vi "Func-엑셀 데이터를 그래프로 출력.vi"() -> ()   [LabVIEW 2015] (continued)
45\t45\t48.154\n45\t45\t48.16\n45\t45\t48.165\n45\t45\t48.164\n45\t45\t48.166\n45\t45\t48.17\n45\t45\t48.174\n45\t45\t48.179\n45\t45\t48.186\n45\t45\t48.187\n45\t45\t48.193\n45\t45\t48.198\n45\t45\t48.202\n45\t45\t48.205\n45\t45\t48.21\n45\t45\t48.216\n45\t45\t48.22\n45\t45\t48.222\n45\t45\t48.229\n45\t45\t48.232\n45\t45\t48.238\n45\t45\t48.24\n45\t45\t48.243\n45\t45\t48.246\n45\t45\t48.248\n45\t45\t48.252\n45\t45\t48.255\n45\t45\t48.258\n45\t45\t48.265\n45\t45\t48.273\n45\t45\t48.283\n45\t45\t48.288\n45\t45\t48.292\n45\t45\t48.296\n45\t45\t48.298\n45\t45\t48.302\n45\t45\t48.299\n45\t45\t48.305\n45\t45\t48.31\n45\t45\t48.314\n45\t45\t48.322\n45\t45\t48.323\n45\t45\t48.325\n45\t45\t48.329\n45\t45\t48.329\n45\t45\t48.334\n45\t45\t48.339\n45\t45\t48.344\n45\t45\t48.352\n45\t45\t48.359\n45\t45\t48.364\n45\t45\t48.366\n45\t45\t48.369\n45\t45\t48.374\n45\t45\t48.375\n45\t45\t48.382\n45\t45\t48.384\n45\t45\t48.39\n45\t45\t48.395\n45\t45\t48.393\n45\t45\t48.397\n45\t45\t48.402\n45\t45\t48.409\n45\t45\t48.417\n45\t45\t48.421\n45\t45\t48.427\n45\t45\t48.431\n45\t45\t48.434\n45\t45\t48.439\n45\t45\t48.441\n45\t45\t48.444\n45\t45\t48.446\n45\t45\t48.449\n45\t45\t48.454\n45\t45\t48.454\n45\t45\t48.46\n45\t45\t48.462\n45\t45\t48.47\n45\t45\t48.479\n45\t45\t48.481\n45\t45\t48.488\n45\t45\t48.491\n45\t45\t48.495\n45\t45\t48.494\n45\t45\t48.495\n45\t45\t48.497\n45\t45\t48.496\n45\t45\t48.503\n45\t45\t48.509\n45\t45\t48.513\n45\t45\t48.518\n45\t45\t48.521\n45\t45\t48.53\n45\t45\t48.531\n45\t45\t48.533\n45\t45\t48.539\n45\t45\t48.543\n45\t45\t48.546\n45\t45\t48.55\n45\t45\t48.552\n45\t45\t48.554\n45\t45\t48.557\n45\t45\t48.562\n45\t45\t48.567\n45\t45\t48.571\n45\t45\t48.577\n45\t45\t48.58\n45\t45\t48.582\n45\t45\t48.59\n45\t45\t48.592\n45\t45\t48.597\n45\t45\t48.596\n45\t45\t48.598\n45\t45\t48.605\n45\t45\t48.605\n45\t45\t48.606\n45\t45\t48.607\n45\t45\t48.617\n45\t45\t48.624\n45\t45\t48.627\n45\t45\t48.631\n45\t45\t48.638\n45\t45\t48.646\n45\t45\t48.646\n45\t45\t48.649\n45\t45\t48.656\n45\t45\t48.66\n45\t45\t48.663\n45\t45\t48.667\n45\t45\t48.673\n45\t45\t48.677\n45\t45\t48.678\n45\t45\t48.68\n45\t45\t48.679\n45\t45\t48.682\n45\t45\t48.683\n45\t45\t48.689\n45\t45\t48.691\n45\t45\t48.694\n45\t45\t48.7\n45\t45\t48.7\n45\t45\t48.703\n45\t45\t48.709\n45\t45\t48.713\n45\t45\t48.716\n45\t45\t48.725\n45\t45\t48.729\n45\t45\t48.732\n45\t45\t48.734\n45\t45\t48.739\n45\t45\t48.743\n45\t45\t48.746\n45\t45\t48.747\n45\t45\t48.753\n45\t45\t48.761\n45\t45\t48.762\n45\t45\t48.767\n45\t45\t48.767\n45\t45\t48.774\n45\t45\t48.779\n45\t45\t48.778\n45\t45\t48.782\n45\t45\t48.789\n45\t45\t48.789\n45\t45\t48.79\n45\t45\t48.793\n45\t45\t48.801\n45\t45\t48.802\n45\t45\t48.808\n45\t45\t48.812\n45\t45\t48.816\n45\t45\t48.82\n45\t45\t48.821\n45\t45\t48.826\n45\t45\t48.825\n45\t45\t48.83\n45\t45\t48.829\n45\t45\t48.829\n45\t45\t48.83\n45\t45\t48.834\n45\t45\t48.837\n45\t45\t48.839\n45\t45\t48.846\n45\t45\t48.853\n45\t45\t48.859\n45\t45\t48.862\n45\t45\t48.869\n45\t45\t48.875\n45\t45\t48.881\n45\t45\t48.882\n45\t45\t48.884\n45\t45\t48.891\n45\t45\t48.89\n45\t45\t48.891\n45\t45\t48.892\n45\t45\t48.895\n45\t45\t48.896\n45\t45\t48.903\n45\t45\t48.905\n45\t45\t48.909\n45\t45\t48.913\n45\t45\t48.92\n45\t45\t48.926\n45\t45\t48.927\n45\t45\t48.931\n45\t45\t48.932\n45\t45\t48.939\n45\t45\t48.939\n45\t45\t48.941\n45\t45\t48.942\n45\t45\t48.949\n45\t45\t48.955\n45\t45\t48.957\n45\t45\t48.963\n45\t45\t48.965\n45\t45\t48.975\n45\t45\t48.979\n45\t45\t48.982\n45\t45\t48.987\n45\t45\t48.988\n45\t45\t48.994\n45\t45\t48.995\n45\t45\t48.991\n45\t45\t48.992\n45\t45\t48.993\n45\t45\t48.996\n45\t45\t48.999\n45\t45\t49.003\n45\t45\t49.007\n45\t45\t49.015\n45\t45\t49.02\n45\t45\t49.025\n45\t45\t49.028\n45\t45\t49.033\n45\t45\t49.036\n45\t45\t49.037\n45\t45\t49.042\n45\t45\t49.045\n45\t45\t49.05\n45\t45\t49.051\n45\t45\t49.055\n45\t45\t49.059\n45\t45\t49.059\n45\t45\t49.057\n45\t45\t49.058\n45\t45\t49.058\n45\t45\t49.061\n45\t45\t49.064\n45\t45\t49.069\n45\t45\t49.073\n45\t45\t49.077\n45\t45\t49.084\n45\t45\t49.086\n45\t45\t49.093\n45\t45\t49.095\n45\t45\t49.101\n45\t45\t49.105\n45\t45\t49.109\n45\t45\t49.111\n45\t45\t49.115\n45\t45\t49.12\n45\t45\t49.12\n45\t45\t49.123\n45\t45\t49.125\n45\t45\t49.131\n45\t45\t49.132\n45\t45\t49.134\n45\t45\t49.139\n45\t45\t49.142\n45\t45\t49.146\n45\t45\t49.148\n45\t45\t49.151\n45\t45\t49.154\n45\t45\t49.159\n45\t45\t49.161\n45\t45\t49.162\n45\t45\t49.165\n45\t45\t49.166\n45\t45\t49.171\n45\t45\t49.173\n45\t45\t49.177\n45\t45\t49.179\n45\t45\t49.184\n45\t45\t49.189\n45\t45\t49.189\n45\t45\t49.195\n45\t45\t49.194\n45\t45\t49.196\n45\t45\t49.199\n45\t45\t49.196\n45\t45\t49.201\n45\t45\t49.204\n45\t45\t49.209\n45\t45\t49.218\n45\t45\t49.221\n45\t45\t49.227\n45\t45\t49.23\n45\t45\t49.232\n45\t45\t49.233\n45\t45\t49.229\n45\t45\t49.232\n45\t45\t49.234\n45\t45\t49.239\n45\t45\t49.241\n45\t45\t49.246\n45\t45\t49.254\n45\t45\t49.256\n45\t45\t49.257\n45\t45\t49.255\n45\t45\t49.259\n45\t45\t49.259\n45\t45\t49.266\n45\t45\t49.27\n45\t45\t49.271\n45\t45\t49.28\n45\t45\t49.282\n45\t45\t49.284\n45\t45\t49.287\n45\t45\t49.29\n45\t45\t49.296\n45\t45\t49.299\n45\t45\t49.301\n45\t45\t49.302\n45\t45\t49.303\n45\t45\t49.305\n45\t45\t49.31\n45\t45\t49.309\n45\t45\t49.311\n45\t45\t49.314\n45\t45\t49.316\n45\t45\t49.316\n45\t45\t49.317\n45\t45\t49.323\n45\t45\t49.327\n45\t45\t49.332\n45\t45\t49.337\n45\t45\t49.34\n45\t45\t49.344\n45\t45\t49.341\n45\t45\t49.343\n45\t45\t49.349\n45\t45\t49.35\n45\t45\t49.352\n45\t45\t49.355\n45\t45\t49.363\n45\t45\t49.365\n45\t45\t49.368\n45\t45\t49.371\n45\t45\t49.375\n45\t45\t49.379\n45\t45\t49.379\n45\t45\t49.384\n45\t45\t49.389\n45\t45\t49.391\n45\t45\t49.393\n45\t45\t49.399\n45\t45\t49.401\n45\t45\t49.405\n45\t45\t49.41\n45\t45\t49.411\n45\t45\t49.413\n45\t45\t49.412\n45\t45\t49.412\n45\t45\t49.413\n45\t45\t49.413\n45\t45\t49.415\n45\t45\t49.419\n45\t45\t49.423\n45\t45\t49.428\n45\t45\t49.433\n45\t45\t49.434\n45\t45\t49.439\n45\t45\t49.44\n45\t45\t49.443\n45\t45\t49.446\n45\t45\t49.45\n45\t45\t49.452\n45\t45\t49.455\n45\t45\t49.463\n45\t45\t49.464\n45\t45\t49.467\n45\t45\t49.466\n45\t45\t49.466\n45\t45\t49.466\n45\t45\t49.471\n45\t45\t49.472\n45\t45\t49.476\n45\t45\t49.479\n45\t45\t49.484\n45\t45\t49.488\n45\t45\t49.489\n45\t45\t49.495\n45\t45\t49.502\n45\t45\t49.507\n45\t45\t49.513\n45\t45\t49.515\n45\t45\t49.517\n45\t45\t49.517\n45\t45\t49.516\n45\t45\t49.517\n45\t45\t49.516\n45\t45\t49.521\n45\t45\t49.524\n45\t45\t49.526\n45\t45\t49.53\n45\t45\t49.531\n45\t45\t49.533\n45\t45\t49.536\n45\t45\t49.541\n45\t45\t49.545\n45\t45\t49.546\n45\t45\t49.552\n45\t45\t49.556\n45\t45\t49.557\n45\t45\t49.554\n45\t45\t49.554\n45\t45\t49.554\n45\t45\t49.555\n45\t45\t49.557\n45\t45\t49.561\n45\t45\t49.564\n45\t45\t49.57\n45\t45\t49.579\n45\t45\t49.582\n45\t45\t49.589\n45\t45\t49.588\n45\t45\t49.593\n45\t45\t49.598\n45\t45\t49.596\n45\t45\t49.599\n45\t45\t49.599\n45\t45\t49.604\n45\t45\t49.6\n45\t45\t49.601\n45\t45\t49.605\n45\t45\t49.605\n45\t45\t49.606\n45\t45\t49.608\n45\t45\t49.614\n45\t45\t49.617\n45\t45\t49.619\n45\t45\t49.623\n45\t45\t49.627\n45\t45\t49.629\n45\t45\t49.629\n45\t45\t49.633\n45\t45\t49.637\n45\t45\t49.638\n45\t45\t49.643\n45\t45\t49.644\n45\t45\t49.647\n45\t45\t49.653\n45\t45\t49.65\n45\t45\t49.654\n45\t45\t49.654\n45\t45\t49.657\n45\t45\t49.662\n45\t45\t49.661\n45\t45\t49.666\n45\t45\t49.664\n45\t45\t49.67\n45\t45\t49.672\n45\t45\t49.677\n45\t45\t49.679\n45\t45\t49.683\n45\t45\t49.689\n45\t45\t49.691\n45\t45\t49.693\n45\t45\t49.699\n45\t45\t49.702\n45\t45\t49.703\n45\t45\t49.705\n45\t45\t49.707\n45\t45\t49.709\n45\t45\t49.711\n45\t45\t49.714\n45\t45\t49.714\n45\t45\t49.716\n45\t45\t49.716\n45\t45\t49.721\n45\t45\t49.72\n45\t45\t49.722\n45\t45\t49.722\n45\t45\t49.725\n45\t45\t49.732\n45\t45\t49.734\n45\t45\t49.737\n45\t45\t49.738\n45\t45\t49.748\n45\t45\t49.75\n45\t45\t49.75\n45\t45\t49.751\n45\t45\t49.753\n45\t45\t49.755\n45\t45\t49.754\n45\t45\t49.756\n45\t45\t49.753\n45\t45\t49.756\n45\t45\t49.759\n45\t45\t49.763\n45\t45\t49.764\n45\t45\t49.767\n45\t45\t49.772\n45\t45\t49.777\n45\t45\t49.779\n45\t45\t49.779\n45\t45\t49.785\n45\t45\t49.788\n45\t45\t49.79\n45\t45\t49.788\n45\t45\t49.792\n45\t45\t49.799\n45\t45\t49.797\n45\t45\t49.799\n45\t45\t49.807\n45\t45\t49.81\n45\t45\t49.809\n45\t45\t49.807\n45\t45\t49.809\n45\t45\t49.81\n45\t45\t49.809\n45\t45\t49.811\n45\t45\t49.816\n45\t45\t49.821\n45\t45\t49.825\n45\t45\t49.828\n45\t45\t49.83\n45\t45\t49.832\n45\t45\t49.833\n45\t45\t49.834\n45\t45\t49.839\n45\t45\t49.84\n45\t45\t49.842\n45\t45\t49.843\n45\t45\t49.847\n45\t45\t49.853\n45\t45\t49.851\n45\t45\t49.854\n45\t45\t49.857\n45\t45\t49.859\n45\t45\t49.857\n45\t45\t49.857\n45\t45\t49.861\n45\t45\t49.864\n45\t45\t49.866\n45\t45\t49.869\n45\t45\t49.871\n45\t45\t49.878\n45\t45\t49.875\n45\t45\t49.878\n45\t45\t49.879\n45\t45\t49.88\n45\t45\t49.885\n45\t45\t49.886\n45\t45\t49.891\n45\t45\t49.893\n45\t45\t49.898\n45\t45\t49.903\n45\t45\t49.909\n45\t45\t49.909\n45\t45\t49.911\n45\t45\t49.916\n45\t45\t49.918\n45\t45\t49.918\n45\t45\t49.92\n45\t45\t49.92\n45\t45\t49.921\n45\t45\t49.92\n45\t45\t49.925\n45\t45\t49.927\n45\t45\t49.928\n45\t45\t49.932\n45\t45\t49.939\n45\t45\t49.943\n45\t45\t49.941\n45\t45\t49.941\n45\t45\t49.943\n45\t45\t49.943\n45\t45\t49.944\n45\t45\t49.945\n45\t45\t49.95\n45\t45\t49.952\n45\t45\t49.954\n45\t45\t49.956\n45\t45\t49.959\n45\t45\t49.96\n45\t45\t49.96\n45\t45\t49.963\n45\t45\t49.963\n45\t45\t49.965\n45\t45\t49.968\n45\t45\t49.97\n45\t45\t49.969\n45\t45\t49.973\n45\t45\t49.979\n45\t45\t49.981\n45\t45\t49.976\n45\t45\t49.98\n45\t45\t49.984\n45\t45\t49.986\n45\t45\t49.986\n45\t45\t49.987\n45\t45\t49.995\n45\t45\t49.992\n45\t45\t49.996\n45\t45\t49.999\n45\t45\t50.003\n45\t45\t50.009\n45\t45\t50.009\n45\t45\t50.013\n45\t45\t50.016\n45\t45\t50.014\n45\t45\t50.015\n45\t45\t50.014\n45\t45\t50.014\n45\t45\t50.017\n45\t45\t50.018\n45\t45\t50.022\n45\t45\t50.021\n45\t45\t50.024\n45\t45\t50.028\n45\t45\t50.029\n45\t45\t50.031\n45\t45\t50.035\n45\t45\t50.04\n45\t45\t50.044\n45\t45\t50.045\n45\t45\t50.049\n45\t45\t50.055\n45\t45\t50.054\n45\t45\t50.058\n45\t45\t50.059\n45\t45\t50.063\n45\t45\t50.066\n45\t45\t50.063\n45\t45\t50.066\n45\t45\t50.068\n45\t45\t50.073\n45\t45\t50.073\n45\t45\t50.074\n45\t45\t50.077\n45\t45\t50.075\n45\t45\t50.076\n45\t45\t50.071\n45\t45\t50.073\n45\t45\t50.073\n45\t45\t50.074\n45\t45\t50.079\n45\t45\t50.078\n45\t45\t50.084\n45\t45\t50.088\n45\t45\t50.09\n45\t45\t50.092\n45\t45\t50.096\n45\t45\t50.101\n45\t45\t50.101\n45\t45\t50.103\n45\t45\t50.105\n45\t45\t50.107\n45\t45\t50.112\n45\t45\t50.11\n45\t45\t50.113\n45\t45\t50.113\n45\t45\t50.117\n45\t45\t50.12\n45\t45\t50.12\n45\t45\t50.121\n45\t45\t50.124\n45\t45\t50.129\n45\t45\t50.129\n45\t45\t50.13\n45\t45\t50.132\n45\t45\t50.134\n45\t45\t50.14\n45\t45\t50.144\n45\t45\t50.146\n45\t45\t50.143\n45\t45\t50.145\n45\t45\t50.149\n45\t45\t50.145\n45\t45\t50.144\n45\t45\t50.146\n45\t45\t50.155\n45\t45\t50.159\n45\t45\t50.159\n45\t45\t50.161\n45\t45\t50.168\n45\t45\t50.17\n45\t45\t50.168\n45\t45\t50.165\n45\t45\t50.17\n45\t45\t50.168\n45\t45\t50.165\n45\t45\t50.167\n45\t45\t50.167\n45\t45\t50.172\n45\t45\t50.172\n45\t45\t50.178\n45\t45\t50.183\n45\t45\t50.187\n45\t45\t50.188\n45\t45\t50.186\n45\t45\t50.19\n45\t45\t50.193\n45\t45\t50.195\n45\t45\t50.198\n45\t45\t50.203\n45\t45\t50.206\n45\t45\t50.204\n45\t45\t50.205\n45\t45\t50.202\n45\t45\t50.199\n45\t45\t50.198\n45\t45\t50.202\n45\t45\t50.206\n45\t45\t50.208\n45\t45\t50.211\n45\t45\t50.218\n45\t45\t50.22\n45\t45\t50.223\n45\t45\t50.223\n45\t45\t50.225\n45\t45\t50.23\n45\t45\t50.228\n45\t45\t50.229\n45\t45\t50.229\n45\t45\t50.233\n45\t45\t50.233\n45\t45\t50.233\n45\t45\t50.234\n45\t45\t50.236\n45\t45\t50.238\n45\t45\t50.24\n45\t45\t50.244\n45\t45\t50.247\n45\t45\t50.25\n45\t45\t50.25\n45\t45\t50.249\n45\t45\t50.246\n45\t45\t50.248\n45\t45\t50.25\n45\t45\t50.252\n45\t45\t50.253\n45\t45\t50.258\n45\t45\t50.263\n45\t45\t50.263\n45\t45\t50.265\n45\t45\t50.269\n45\t45\t50.27\n45\t45\t50.271\n45\t45\t50.272\n45\t45\t50.272\n45\t45\t50.273\n45\t45\t50.274\n45\t45\t50.279\n45\t45\t50.279\n45\t45\t50.28\n45\t45\t50.286\n45\t45\t50.287\n45\t45\t50.287\n45\t45\t50.288\n45\t45\t50.291\n45\t45\t50.294\n45\t45\t50.295\n45\t45\t50.298\n45\t45\t50.303\n45\t45\t50.31\n45\t45\t50.313\n45\t45\t50.313\n45\t45\t50.314\n45\t45\t50.318\n45\t45\t50.318\n45\t45\t50.315\n45\t45\t50.314\n45\t45\t50.32\n45\t45\t50.322\n45\t45\t50.318\n45\t45\t50.32\n45\t45\t50.323\n45\t45\t50.324\n45\t45\t50.322\n45\t45\t50.322\n45\t45\t50.327\n45\t45\t50.326\n45\t45\t50.327\n45\t45\t50.332\n45\t45\t50.338\n45\t45\t50.339\n45\t45\t50.338\n45\t45\t50.346\n45\t45\t50.35\n45\t45\t50.348\n45\t45\t50.347\n45\t45\t50.352\n45\t45\t50.355\n45\t45\t50.358\n45\t45\t50.357\n45\t45\t50.354\n45\t45\t50.36\n45\t45\t50.359\n45\t45\t50.36\n45\t45\t50.358\n45\t45\t50.364\n45\t45\t50.365\n45\t45\t50.368\n45\t45\t50.372\n45\t45\t50.376\n45\t45\t50.373\n45\t45\t50.371\n45\t45\t50.372\n45\t45\t50.372\n45\t45\t50.37\n45\t45\t50.375\n45\t45\t50.377\n45\t45\t50.379\n45\t45\t50.382\n45\t45\t50.386\n45\t45\t50.391\n45\t45\t50.39\n45\t45\t50.395\n45\t45\t50.395\n45\t45\t50.398\n45\t45\t50.395\n45\t45\t50.394\n45\t45\t50.395\n45\t45\t50.393\n45\t45\t50.396\n45\t45\t50.402\n45\t45\t50.407\n45\t45\t50.405\n45\t45\t50.409\n45\t45\t50.414\n45\t45\t50.414\n45\t45\t50.409\n45\t45\t50.408\n45\t45\t50.413\n45\t45\t50.416\n45\t45\t50.417\n45\t45\t50.421\n45\t45\t50.427\n45\t45\t50.431\n45\t45\t50.427\n45\t45\t50.428\n45\t45\t50.428\n45\t45\t50.43\n45\t45\t50.43\n45\t45\t50.426\n45\t45\t50.432\n45\t45\t50.432\n45\t45\t50.434\n45\t45\t50.432\n45\t45\t50.433\n45\t45\t50.437\n45\t45\t50.438\n45\t45\t50.44\n45\t45\t50.438\n45\t45\t50.446\n45\t45\t50.448\n45\t45\t50.453\n45\t45\t50.452\n45\t45\t50.451\n45\t45\t50.454\n45\t45\t50.45\n45\t45\t50.451\n45\t45\t50.453\n45\t45\t50.454\n45\t45\t50.453\n45\t45\t50.456\n45\t45\t50.461\n45\t45\t50.463\n45\t45\t50.462\n45\t45\t50.465\n45\t45\t50.469\n45\t45\t50.473\n45\t45\t50.472\n45\t45\t50.476\n45\t45\t50.479\n45\t45\t50.486\n45\t45\t50.485\n45\t45\t50.482\n45\t45\t50.484\n45\t45\t50.485\n45\t45\t50.486\n45\t45\t50.483\n45\t45\t50.488\n45\t45\t50.493\n45\t45\t50.496\n45\t45\t50.494\n45\t45\t50.496\n45\t45\t50.496\n45\t45\t50.5\n45\t45\t50.5\n45\t45\t50.497\n45\t45\t50.498\n45\t45\t50.502\n45\t45\t50.504\n45\t45\t50.505\n45\t45\t50.509\n45\t45\t50.514\n45\t45\t50.515\n45\t45\t50.514\n45\t45\t50.512\n45\t45\t50.51\n45\t45\t50.509\n45\t45\t50.509\n45\t45\t50.511\n45\t45\t50.509\n45\t45\t50.514\n45\t45\t50.523\n45\t45\t50.522\n45\t45\t50.524\n45\t45\t50.527\n45\t45\t50.534\n45\t45\t50.532\n45\t45\t50.527\n45\t45\t50.532\n45\t45\t50.534\n45\t45\t50.538\n45\t45\t50.537\n45\t45\t50.541\n45\t45\t50.545\n45\t45\t50.546\n45\t45\t50.544\n45\t45\t50.542\n45\t45\t50.543\n45\t45\t50.542\n45\t45\t50.543\n45\t45\t50.543\n45\t45\t50.551\n45\t45\t50.554\n45\t45\t50.557\n45\t45\t50.557\n45\t45\t50.557\n45\t45\t50.557\n45\t45\t50.555\n45\t45\t50.56\n45\t45\t50.559\n45\t45\t50.564\n45\t45\t50.564\n45\t45\t50.566\n45\t45\t50.569\n45\t45\t50.565\n45\t45\t50.566\n45\t45\t50.567\n45\t45\t50.571\n45\t45\t50.575\n45\t45\t50.575\n45\t45\t50.575\n45\t45\t50.576\n45\t45\t50.577\n45\t45\t50.577\n45\t45\t50.578\n45\t45\t50.58\n45\t45\t50.582\n45\t45\t50.583\n45\t45\t50.587\n45\t45\t50.586\n45\t45\t50.588\n45\t45\t50.588\n45\t45\t50.591\n45\t45\t50.593\n45\t45\t50.594\n45\t45\t50.596\n45\t45\t50.599\n45\t45\t50.604\n45\t45\t50.606\n45\t45\t50.608\n45\t45\t50.61\n45\t45\t50.609\n45\t45\t50.606\n45\t45\t50.604\n45\t45\t50.604\n45\t45\t50.607\n45\t45\t50.609\n45\t45\t50.615\n45\t45\t50.617\n45\t45\t50.617\n45\t45\t50.618\n45\t45\t50.616\n45\t45\t50.615\n45\t45\t50.618\n45\t45\t50.623\n45\t45\t50.624\n45\t45\t50.623\n45\t45\t50.626\n45\t45\t50.626\n45\t45\t50.622\n45\t45\t50.622\n45\t45\t50.626\n45\t45\t50.628\n45\t45\t50.63\n45\t45\t50.634\n45\t45\t50.639\n45\t45\t50.638\n45\t45\t50.635\n45\t45\t50.64\n45\t45\t50.64\n45\t45\t50.642\n45\t45\t50.641\n45\t45\t50.645\n45\t45\t50.648\n45\t45\t50.65\n45\t45\t50.651\n45\t45\t50.648\n45\t45\t50.646\n45\t45\t50.647\n45\t45\t50.647\n45\t45\t50.645\n45\t45\t50.649\n45\t45\t50.65\n45\t45\t50.654\n45\t45\t50.656\n45\t45\t50.662\n45\t45\t50.663\n45\t45\t50.664\n45\t45\t50.661\n45\t45\t50.664\n45\t45\t50.665\n45\t45\t50.665\n45\t45\t50.666\n45\t45\t50.664\n45\t45\t50.667\n45\t45\t50.666\n45\t45\t50.668\n45\t45\t50.672\n45\t45\t50.675\n45\t45\t50.68\n45\t45\t50.686\n45\t45\t50.685\n45\t45\t50.683\n45\t45\t50.682\n45\t45\t50.683\n45\t45\t50.683\n45\t45\t50.684\n45\t45\t50.687\n45\t45\t50.693\n45\t45\t50.691\n45\t45\t50.693\n45\t45\t50.694\n45\t45\t50.695\n45\t45\t50.693\n45\t45\t50.692\n45\t45\t50.697\n45\t45\t50.696\n45\t45\t50.696\n45\t45\t50.696\n45\t45\t50.701\n45\t45\t50.703\n45\t45\t50.702\n45\t45\t50.708\n45\t45\t50.71\n45\t45\t50.715\n45\t45\t50.718\n45\t45\t50.721\n45\t45\t50.722\n45\t45\t50.722\n45\t45\t50.724\n45\t45\t50.721\n45\t45\t50.718\n45\t45\t50.717\n45\t45\t50.718\n45\t45\t50.718\n45\t45\t50.721\n45\t45\t50.722\n45\t45\t50.725\n45\t45\t50.73\n45\t45\t50.733\n45\t45\t50.736\n45\t45\t50.735\n45\t45\t50.739\n45\t45\t50.739\n45\t45\t50.74\n45\t45\t50.736\n45\t45\t50.737\n45\t45\t50.741\n45\t45\t50.741\n45\t45\t50.742\n45\t45\t50.742\n45\t45\t50.746\n45\t45\t50.746\n45\t45\t50.745\n45\t45\t50.747\n45\t45\t50.748\n45\t45\t50.749\n45\t45\t50.752\n45\t45\t50.755\n45\t45\t50.755\n45\t45\t50.756\n45\t45\t50.759\n45\t45\t50.759\n45\t45\t50.76\n45\t45\t50.757\n45\t45\t50.759\n45\t45\t50.761\n45\t45\t50.761\n45\t45\t50.765\n45\t45\t50.764\n45\t45\t50.766\n45\t45\t50.771\n45\t45\t50.77\n45\t45\t50.771\n45\t45\t50.768\n45\t45\t50.77\n45\t45\t50.771\n45\t45\t50.769\n45\t45\t50.772\n45\t45\t50.772\n45\t45\t50.775\n45\t45\t50.775\n45\t45\t50.772\n45\t45\t50.773\n45\t45\t50.773\n45\t45\t50.774\n45\t45\t50.773\n45\t45\t50.775\n45\t45\t50.78\n45\t45\t50.784\n45\t45\t50.786\n45\t45\t50.789\n45\t45\t50.792\n45\t45\t50.795\n45\t45\t50.795\n45\t45\t50.791\n45\t45\t50.791\n45\t45\t50.794\n45\t45\t50.796\n45\t45\t50.796\n45\t45\t50.797\n45\t45\t50.802\n45\t45\t50.802\n45\t45\t50.8\n45\t45\t50.802\n45\t45\t50.803\n45\t45\t50.807\n45\t45\t50.806\n45\t45\t50.806\n45\t45\t50.804\n45\t45\t50.805\n45\t45\t50.807\n45\t45\t50.805\n45\t45\t50.805\n45\t45\t50.808\n45\t45\t50.812\n45\t45\t50.814\n45\t45\t50.812\n45\t45\t50.816\n45\t45\t50.818\n45\t45\t50.818\n45\t45\t50.817\n45\t45\t50.819\n45\t45\t50.82\n45\t45\t50.819\n45\t45\t50.82\n45\t45\t50.826\n45\t45\t50.829\n45\t45\t50.825\n45\t45\t50.827\n45\t45\t50.834\n45\t45\t50.836\n45\t45\t50.835\n45\t45\t50.835\n45\t45\t50.837\n45\t45\t50.836\n45\t45\t50.832\n45\t45\t50.829\n45\t45\t50.827\n45\t45\t50.83\n45\t45\t50.833\n45\t45\t50.834\n45\t45\t50.837\n45\t45\t50.843\n45\t45\t50.844\n45\t45\t50.842\n45\t45\t50.843\n45\t45\t50.848\n45\t45\t50.848\n45\t45\t50.844\n45\t45\t50.848\n45\t45\t50.85\n45\t45\t50.847\n45\t45\t50.846\n45\t45\t50.846\n45\t45\t50.85\n45\t45\t50.85\n45\t45\t50.85\n45\t45\t50.851\n45\t45\t50.855\n45\t45\t50.856\n45\t45\t50.858\n45\t45\t50.86\n45\t45\t50.863\n45\t45\t50.867\n45\t45\t50.866\n45\t45\t50.866\n45\t45\t50.869\n45\t45\t50.867\n45\t45\t50.866\n45\t45\t50.868\n45\t45\t50.87\n45\t45\t50.872\n45\t45\t50.866\n45\t45\t50.867\n45\t45\t50.868\n45\t45\t50.868\n45\t45\t50.864\n45\t45\t50.866\n45\t45\t50.87\n45\t45\t50.869\n45\t45\t50.871\n45\t45\t50.871\n45\t45\t50.876\n45\t45\t50.879\n45\t45\t50.88\n45\t45\t50.884\n45\t45\t50.884\n45\t45\t50.887\n45\t45\t50.891\n45\t45\t50.892\n45\t45\t50.896\n45\t45\t50.896\n45\t45\t50.9\n45\t45\t50.903\n45\t45\t50.898\n45\t45\t50.897\n45\t45\t50.893\n45\t45\t50.899\n45\t45\t50.898\n45\t45\t50.898\n45\t45\t50.902\n45\t45\t50.905\n45\t45\t50.907\n45\t45\t50.903\n45\t45\t50.901\n45\t45\t50.901\n45\t45\t50.897\n45\t45\t50.896\n45\t45\t50.895\n45\t45\t50.896\n45\t45\t50.899\n45\t45\t50.9\n45\t45\t50.908\n45\t45\t50.909\n45\t45\t50.914\n45\t45\t50.916\n45\t45\t50.916\n45\t45\t50.916\n45\t45\t50.915\n45\t45\t50.919\n45\t45\t50.919\n45\t45\t50.917\n45\t45\t50.916\n45\t45\t50.918\n45\t45\t50.92\n45\t45\t50.918\n45\t45\t50.92\n45\t45\t50.92\n45\t45\t50.924\n45\t45\t50.926\n45\t45\t
